vi "7_Time_solution.vi"(11 "Seconds":string) -> (1 "Seconds":u32, 2 "Minutes":u32, 3 "Hours":u32)   [LabVIEW 2014]
panel:
  # "Tranfrom seconds into hours/minutes/seconds\nexample\n3800 seconds = 1 Hour 3 Minutes and 20 Seconds"
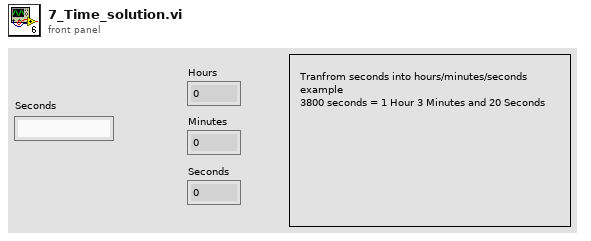
[diagram p1: front panel]
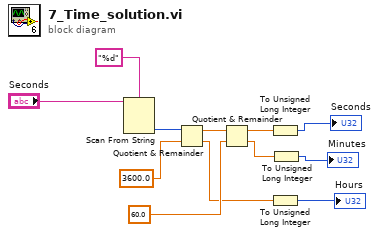
[diagram p0: block diagram]
diagram:
  n1 = Scan From String(format string="%d", input string="Seconds") -> (output 1=w10:i32)  [unwired: 3 in, 3 out]
  n2 = Quotient & Remainder(x=w10, y=3600.0) -> (x-y*floor(x/y)=w8:dbl, floor(x/y)=w3:dbl)
  n3 = Quotient & Remainder(x=w8, y=60.0) -> (x-y*floor(x/y)=w6:dbl, floor(x/y)=w5:dbl)
  n4 = To Unsigned Long Integer(number=w6) -> (unsigned 32bit integer=→"Seconds":u32)
  n5 = To Unsigned Long Integer(number=w3) -> (unsigned 32bit integer=→"Hours":u32)
  n6 = To Unsigned Long Integer(number=w5) -> (unsigned 32bit integer=→"Minutes":u32)
